vi "component_specification_to_URI.vi"(8 "error in (no error)":errorcluster, 10 "component specification":T1) -> (0 "error out":errorcluster, 2 "URI":string)   [LabVIEW 2011, in "StreamingBase.lvclass"]
uses:
  StreamingBase.lvclass
  component_specification_cluster.ctl
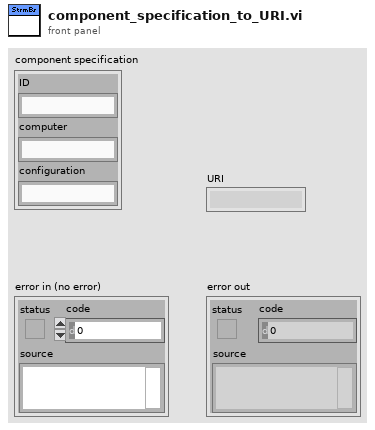
[diagram p1: front panel]
types:
  T1 = typedef "StreamingBase.lvclass/component_specification_cluster.ctl" = cluster{"ID":string, "computer":string, "configuration":string}
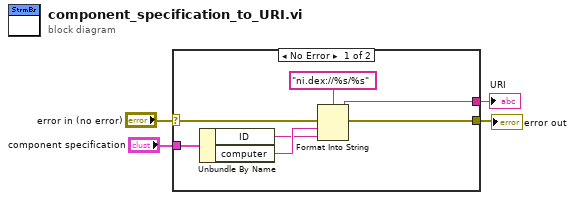
[diagram p0: block diagram]
diagram:
  n1 = case shown="No Error" "error in (no error)" {
    selector: "error in (no error)" -> [w10 w12]
    tunnel: "component specification" -> [w11 _]
    tunnel: [w6 w12] -> w2
    tunnel: [w5 _] -> w1
    frame No Error {
      n2 = Unbundle By Name(w11) -> ("ID"=w7:string, "computer"=w8:string)
      n3 = Format Into String(format string="ni.dex://%s/%s", error in=w10, w8, w7) -> (resulting string=w5:string, error out=w6:errorcluster)  [unwired: 1 in]
    }
    frame Error {
    }
  }
  "error out" <- w2
  "URI" <- w1
